vi "Overlay_Lichtgitterposition.vi"(8 "error in":errorcluster, 10 "Durchmesser Kontakt":dbl, 11 "Cluster in":T1={"Initialisierung"={"Online?"=FALSE, "Grundpfad"=path "", "Kamera Oben"="", "IP-Adresse Flüssiglinse"="", "Flüssiglinse"=refnum, "Kamera Unten"="", "IP-Adresse SPS"="", "SPS-Verbindung"={"TCP Connection Ref"=refnum, "IP address"="", "timeout ms"=5000, "Connected?"=FALSE, "PLC Type"=enum."S7 1200", "Rack S7 400"=0, "Slot S7 400"=0, "PDU Size"=0, "connection semaphore"=refnum}, "IP-Adresse Lichtgitter"="", "Lichtgitter"=refnum, "Skalierungsfaktor x"=0.0, "Skalierungsfaktor y"=0.0, "Bilder Oben"=[], "Bild Unten"=refnum}, "Einstellungen"={"i. O. Bilder speichern"=FALSE, "Ausgewähltes Offline-Datum"="", "Ausgewähltes Offline-Teil"="", "Speicherpfad Bilder"=path "", "Kontakt nicht inkrementieren?"=FALSE}, "Artikeldaten"={"Artikelnummer"="", "Fertigungsauftrag"="", "Belichtungszeit Referenzmarken"=0.0, "Fokus Referenzmarken"=0.0, "Belichtungszeit ISO"=0.0, "Fokus ISO"=0.0, "Belichtungszeit Kontakte"=0.0, "Fokus Kontakte"=0.0, "Belichtungszeit Unten"=0.0, "Kontaktanzahl"=0, "Aktueller Kontakt"=0, "Kontaktposition"={"x"=0.0, "y"=0.0}}, "Kamera Oben"={"Koordinatensystem"={"Punkt x-Achse"={"X"=0.0, "Y"=0.0}, "Uhrsprung"={"X"=0.0, "Y"=0.0}, "Punkt y-Achse"={"X"=0.0, "Y"=0.0}}, "Position Kontakt"={"x"=0.0, "y"=0.0}, "Winkel Kontakt"=0.0, "Referenzen & Kontakt gefunden?"=FALSE, "Prüfung Oben i. O."=FALSE}, "Kamera Unten"={"Prüfung Unten i. O."=FALSE}, "Messung Lichtgitter"={"Kontakt & WT in Lichtgitter?"=FALSE, "Aktuelle Messwerte"=[], "Offset"={"x"=0.0, "y"=0.0}}, "Statistik"={"Statistiken"=[]}}) -> (0 "error out":errorcluster)   [LabVIEW 2024]
uses:
  Typdefinitionen/Cluster.ctl
  <vilib>/userDefined/High Color/IMAQdx.ctl
  <vilib>/DATA AHEAD/SP7/typedefs/S7 Connection.ctl
  <vilib>/DATA AHEAD/SP7/typedefs/PLC Type.ctl
  <vilib>/vision/Image Controls.llb/IMAQ Image.ctl
  Typdefinitionen/Koordinatensystem.ctl
  Typdefinitionen/Statistik.ctl
  <vilib>/Analysis/Matrix/Numeric/Multiply/Multiply - RM,RM.vi
  <vilib>/Analysis/Matrix/Numeric/Conversions/Matrix To Array - RM.vi
  <vilib>/Analysis/Matrix/NI_Matrix.lvlib
  <vilib>/vision/NI_Vision_Development_Module.lvlib
  <vilib>/DATA AHEAD/SP7/SP7.lvlib
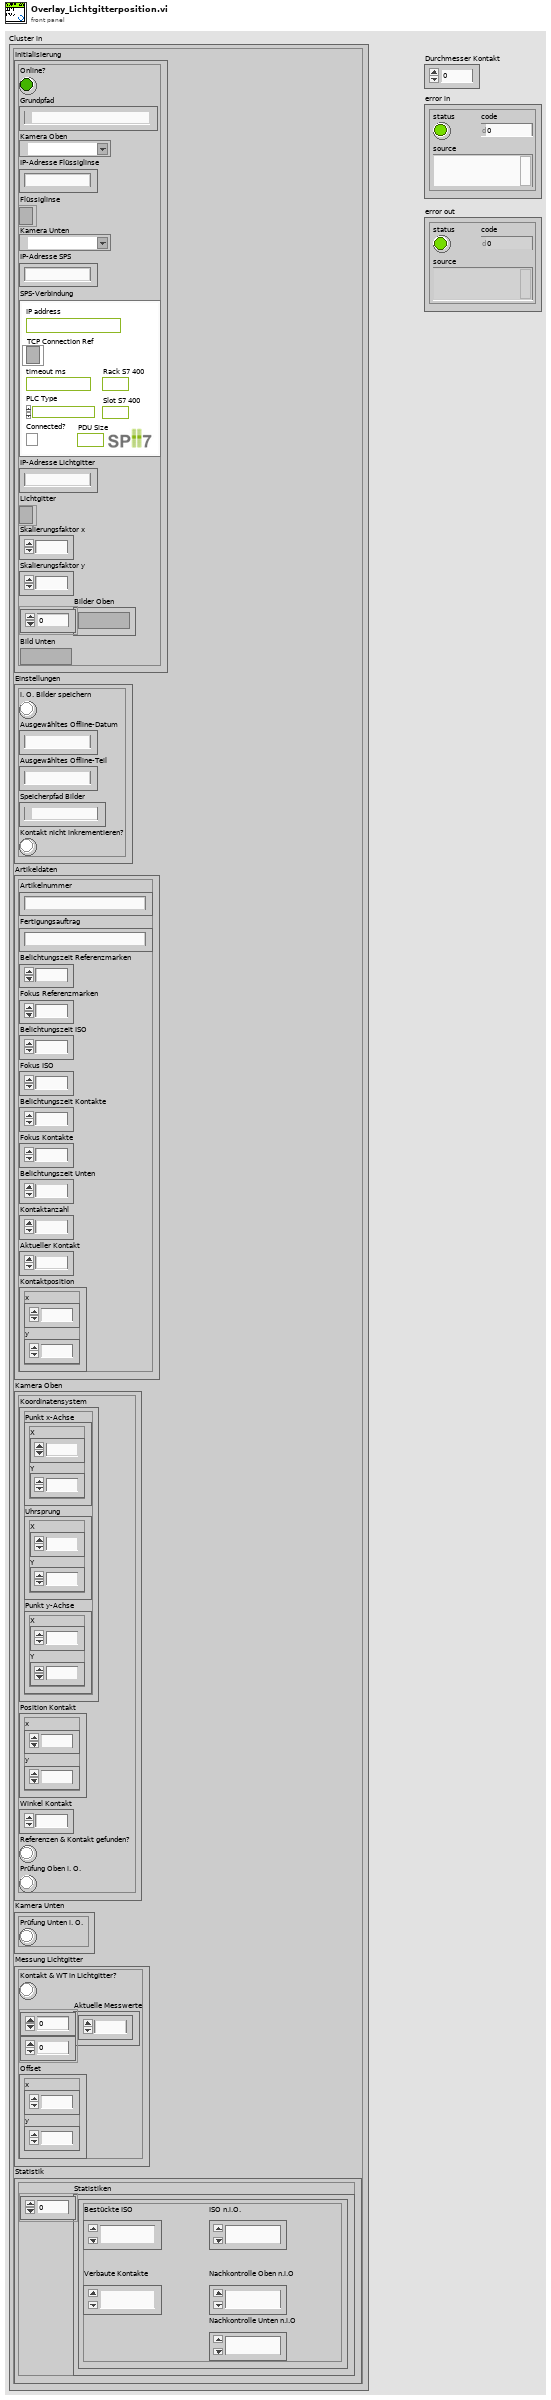
[diagram p1: front panel]
types:
  T1 = typedef "Cluster.ctl" = cluster{"Initialisierung":cluster{"Online?":bool, "Grundpfad":path, "Kamera Oben":T2, "IP-Adresse Flüssiglinse":string, "Flüssiglinse":refnum<k5>, "Kamera Unten":T2, "IP-Adresse SPS":string, "SPS-Verbindung":T3, "IP-Adresse Lichtgitter":string, "Lichtgitter":refnum<k5>, "Skalierungsfaktor x":dbl, "Skalierungsfaktor y":dbl, "Bilder Oben":T6[], "Bild Unten":T6}, "Einstellungen":cluster{"i. O. Bilder speichern":bool, "Ausgewähltes Offline-Datum":string, "Ausgewähltes Offline-Teil":string, "Speicherpfad Bilder":path, "Kontakt nicht inkrementieren?":bool}, "Artikeldaten":cluster{"Artikelnummer":string, "Fertigungsauftrag":string, "Belichtungszeit Referenzmarken":dbl, "Fokus Referenzmarken":dbl, "Belichtungszeit ISO":dbl, "Fokus ISO":dbl, "Belichtungszeit Kontakte":dbl, "Fokus Kontakte":dbl, "Belichtungszeit Unten":dbl, "Kontaktanzahl":u32, "Aktueller Kontakt":i16, "Kontaktposition":cluster{"x":sgl, "y":sgl}}, "Kamera Oben":cluster{"Koordinatensystem":T7, "Position Kontakt":cluster{"x":dbl, "y":dbl}, "Winkel Kontakt":dbl, "Referenzen & Kontakt gefunden?":bool, "Prüfung Oben i. O.":bool}, "Kamera Unten":cluster{"Prüfung Unten i. O.":bool}, "Messung Lichtgitter":cluster{"Kontakt & WT in Lichtgitter?":bool, "Aktuelle Messwerte":dbl[][], "Offset":cluster{"x":dbl, "y":dbl}}, "Statistik":cluster{"Statistiken":T8[]}}
  T2 = typedef "IMAQdx.ctl" = refnum<k21>
  T3 = typedef "SP7.lvlib/S7 Connection.ctl" = cluster{"TCP Connection Ref":refnum<k5>, "IP address":string, "timeout ms":i32, "Connected?":bool, "PLC Type":T4, "Rack S7 400":u8, "Slot S7 400":u8, "PDU Size":u16, "connection semaphore":T5}
  T4 = typedef "SP7.lvlib/PLC Type.ctl" = enum16{"S7 200", "S7 300/400", "S7 1200", "S7 1500", "LOGO!8"}
  T5 = typedef "Semaphore RefNum" = refnum<k1>
  T6 = typedef "IMAQ Image.ctl" = refnum<image>
  T7 = typedef "Koordinatensystem.ctl" = cluster{"Punkt x-Achse":cluster{"X":sgl, "Y":sgl}, "Uhrsprung":cluster{"X":sgl, "Y":sgl}, "Punkt y-Achse":cluster{"X":sgl, "Y":sgl}}
  T8 = typedef "Statistik.ctl" = cluster{"Bestückte ISO":u32, "Verbaute Kontakte":u32, "ISO n.i.O.":u32, "Nachkontrolle Oben n.i.O":u32, "Nachkontrolle Unten n.i.O":u32}
  T9 = cluster{"Position":cluster{"X":sgl, "Y":sgl}, "Radius":dbl, "Score":dbl}
  T10 = cluster{"Farbe Kreis":u32, "Kreis ausfüllen?":bool, "Bounding Rechteck anzeigen?":bool, "Farbe Bounding Rechteck":u32}
  T11 = typedef "NI_Matrix.lvlib/RealMatrix.ctl" = dbl[][]
  T12 = cluster{"Position":cluster{"X":sgl, "Y":sgl}, "Radius":dbl, "Score":dbl}[]
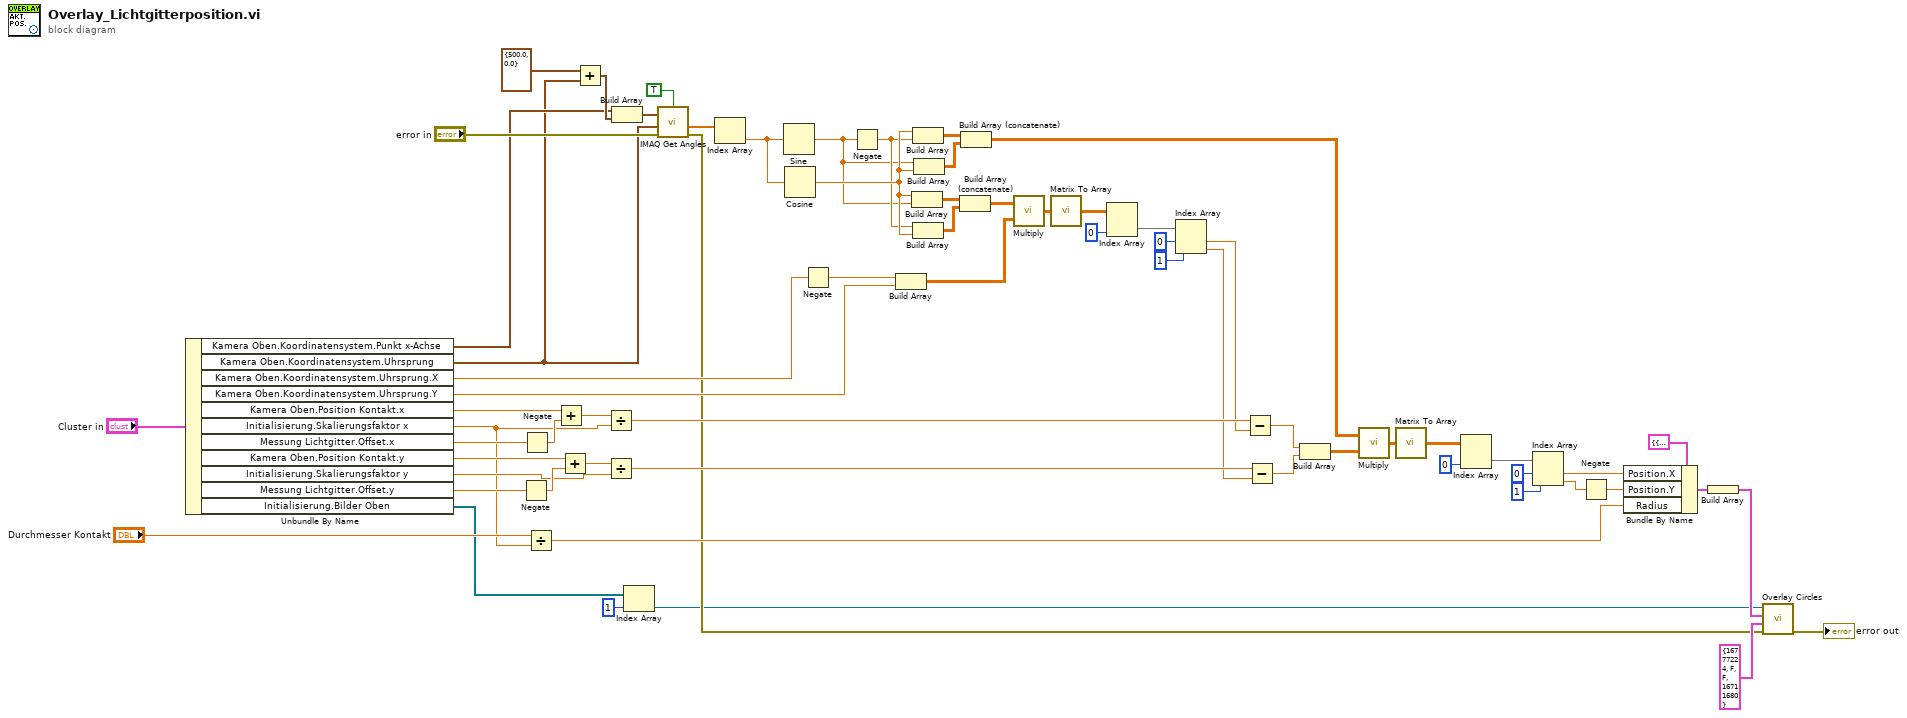
[diagram p0: block diagram]
diagram:
  n1 = Unbundle By Name("Cluster in") -> ("Kamera Oben.Koordinatensystem.Punkt x-Achse"=w50:cluster{"X":sgl, "Y":sgl}, "Kamera Oben.Koordinatensystem.Uhrsprung"=w49:cluster{"X":sgl, "Y":sgl}, "Kamera Oben.Koordinatensystem.Uhrsprung.X"=w12:sgl, "Kamera Oben.Koordinatensystem.Uhrsprung.Y"=w25:sgl, "Kamera Oben.Position Kontakt.x"=w40:dbl, "Initialisierung.Skalierungsfaktor x"=w33:dbl, "Messung Lichtgitter.Offset.x"=w42:dbl, "Kamera Oben.Position Kontakt.y"=w37:dbl, "Initialisierung.Skalierungsfaktor y"=w34:dbl, "Messung Lichtgitter.Offset.y"=w41:dbl, "Initialisierung.Bilder Oben"=w43:T6[])
  n2 = Negate(x=w41) -> (-x=w38:dbl)
  n3 = Negate(x=w42) -> (-x=w39:dbl)
  n4 = Divide(x="Durchmesser Kontakt", y=w33) -> (x/y=w53:dbl)
  n5 = Add(x=w40, y=w39) -> (x+y=w36:dbl)
  n6 = Add(x=w37, y=w38) -> (x+y=w35:dbl)
  n7 = Add(x=cluster{"X":sgl, "Y":sgl} {"X"=500.0, "Y"=0.0} ("y"), y=w49) -> (x+y=w51:cluster{"X":sgl, "Y":sgl})
  n8 = Divide(x=w36, y=w33) -> (x/y=w21:dbl)
  n9 = Divide(x=w35, y=w34) -> (x/y=w18:dbl)
  n10 = Build Array(w50, w51) -> (w55:cluster{"X":sgl, "Y":sgl}[])
  n11 = Index Array(array=w43, index=1) -> (element=w2:T6)
  n12 = call "IMAQ Get Angles"("error in (no error)"="error in", "Vertex"=w49, "Points"=w55, "Use Vertex (No)"=TRUE) -> ("error out"=w3:errorcluster, "Angles (rad)"=w22:sgl[])  [unwired: 1 in, 1 out]
  n13 = Index Array(array=w22) -> (element=w48:sgl)  [unwired: 1 in]
  n14 = Sine(x=w48) -> (sin(x)=w7:sgl)
  n15 = Cosine(x=w48) -> (cos(x)=w14:sgl)
  n16 = Negate(x=w12) -> (-x=w11:sgl)
  n17 = Negate(x=w7) -> (-x=w8:sgl)
  n18 = Build Array(w11, w25) -> (w13:T11)
  n19 = Build Array(w14, w7) -> (w29:T11)
  n20 = Build Array(w14, w8) -> (w58:T11)
  n21 = Build Array(w8, w14) -> (w30:T11)
  n22 = Build Array(w7, w14) -> (w57:T11)
  n23 = Build Array (concatenate)(w29, w30) -> (w9:T11)
  n24 = Build Array (concatenate)(w58, w57) -> (w6:T11)
  n25 = call-poly <vilib>:"Multiply.vi"("Real Matrix B"=w13, "Real Matrix A"=w9) -> ("A * B"=w27:T11)
  n26 = call-poly <vilib>:"Matrix To Array.vi"("Real Matrix"=w27) -> ("Real 2D Array"=w26:dbl[][])
  n27 = Index Array(array=w26, index (col)=0 ("disabled index (col)")) -> (element=w15:dbl[])  [unwired: 1 in]
  n28 = Index Array(array=w15, index #1=0 ("index"), index #2=1 ("index")) -> (element #1=w20:dbl, element #2=w17:dbl)
  n29 = Subtract(x=w21, y=w20) -> (x-y=w19:dbl)
  n30 = Subtract(x=w18, y=w17) -> (x-y=w16:dbl)
  n31 = Build Array(w19, w16) -> (w31:T11)
  n32 = call-poly <vilib>:"Multiply.vi"("Real Matrix B"=w31, "Real Matrix A"=w6) -> ("A * B"=w59:T11)
  n33 = call-poly <vilib>:"Matrix To Array.vi"("Real Matrix"=w59) -> ("Real 2D Array"=w60:dbl[][])
  n34 = Index Array(array=w60, index (col)=0 ("disabled index (col)")) -> (element=w10:dbl[])  [unwired: 1 in]
  n35 = Index Array(array=w10, index #1=0 ("index"), index #2=1 ("index")) -> (element #1=w64:dbl, element #2=w4:dbl)
  n36 = Negate(x=w4) -> (-x=w5:dbl)
  n37 = Bundle By Name(cluster=T9 {"Position"={"X"=0.0, "Y"=0.0}, "Radius"=0.0, "Score"=0.0} ("Circle Descriptor"), "Position.X"=w64, "Position.Y"=w5, "Radius"=w53) -> (w45:T9)
  n38 = Build Array(w45) -> (w66:T12)
  n39 = call "Overlay Circles.vi"("error in"=w3, "Einstellungen"=T10 {"Farbe Kreis"=16777224, "Kreis ausfüllen?"=FALSE, "Bounding Rechteck anzeigen?"=FALSE, "Farbe Bounding Rechteck"=16711680}, "Circles"=w66, "Image in"=w2) -> ("error out"=→"error out":errorcluster)  [unwired: 6 in, 1 out]
